vi "DSF.Engine.Memory.Cache.Transfer Group.Get Transfer Caches.vi"(8 "error in (no error)":errorcluster, 11 "Transfer Group Cache in":refnum<class "DSF.Engine.Memory.Cache.Transfer Group.lvclass">) -> (0 "error out":errorcluster, 2 "Transfer Caches":refnum<class "DSF.Engine.Memory.Cache.Transfer.lvclass">[](array[class]), 3 "Transfer Group Cache out":refnum<class "DSF.Engine.Memory.Cache.Transfer Group.lvclass">)   [LabVIEW 2016, in "DSF.Engine.lvlib" / "DSF.Engine.Memory.Cache.Transfer Group.lvclass"]
uses:
  DSF.Engine.Memory.Cache.Transfer Group.lvclass
  DSF.Engine.Memory.Cache.Transfer.lvclass
  DSF.Engine.Memory.Cache.Transfer Group.lvclass/DSF.Engine.Memory.Cache.Transfer Group.ctl
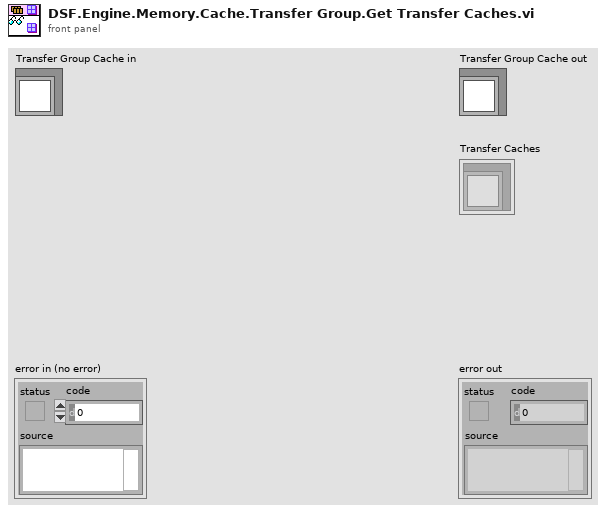
[diagram p1: front panel]
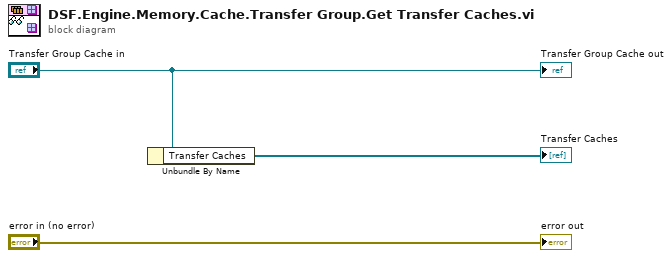
[diagram p0: block diagram]
diagram:
  n1 = Unbundle By Name("Transfer Group Cache in") -> ("Transfer Caches"=→"Transfer Caches":refnum<class "DSF.Engine.Memory.Cache.Transfer.lvclass">[])
  "error out" <- "error in (no error)"
  "Transfer Group Cache out" <- "Transfer Group Cache in"
